vi "CPP-Multiplot.vi"(0 "PlotArray":cluster{dbl[], dbl[]}[](array[cluster]), 1 "Job Directory":path) -> (2 "Saved Automatically?":bool, 3 "gnuplotScript":string, 4 "Plot data file":path)   [LabVIEW 2013]
uses:
  gnuplotScriptComponents/plotstyle.ctl
  gnuplotScriptComponents/graphPeripherals.ctl
  gnuplotScriptComponents/minAndMax.ctl
  gnuplotScriptComponents/AutoManualNumber.ctl
  gnuplotScriptComponents/ticsAndGrids.ctl
  gnuplotScriptComponents/tics.ctl
  gnuplotScriptComponents/grids.ctl
  gnuplotScriptComponents/legendProperties.ctl
  gnuplotScriptComponents/legendAppearance.ctl
  gnuplotScriptComponents/alignment.ctl
  gnuplotScriptComponents/at.ctl
  gnuplotScriptComponents/margins.ctl
  gnuplotScriptComponents/source.ctl
  gnuplotScriptComponents/Master_Legend.ctl
  gnuplotScriptComponents/MasterPeripherals.ctl
  gnuplotScriptComponents/axisName.ctl
  Results_plotter_Global.vi
panel:
  in  "OpenLogfile?":bool
  in  "Show Script Editor?":bool
  in  "Tab Control":T1(tab)=enum."Appearance"
  in  "Each Graph contains:":T2=enum."Series"
  in  "Rows from:":T2=enum."Until done"
  in  "Columns from:":T2=enum."Selector 1"
  in  "Margins":T3={"Top"=2.0, "Bottom"=2.0, "Left"=2.0, "Right"=2.0}
  in  "Height (in)":dbl=7.0 min=0.5 step=0.5 format="%.1f"
  in  "Width (in)":dbl=10.0 min=0.5 step=0.5 format="%.1f"
  in  "nRows":u8=3 min=1
  in  "nCols":u8=3 min=1
  in  "ScaleAdjust":dbl=0.9 min=0.1 max=2.0 step=0.1
  in  "ManualPlotTitles":string[](array[string])
  out "AutoPlotTitles":string[](array[string])
  in  "Individual Plot Titles":bool=TRUE
  in  "Page Title Pre Block":string
  in  "Page Title Post Block":string
  in  "Values to include in Page Title":i32[](listbox)
  in  "Plot Title Offset (characters)":cluster{"horizontal":dbl, "vertical":dbl}
  out "Final Title":string
  in  "Plot Legends Manual":string[](array[string])
  in  "Plotstyles":T4[](array[typedef])=[{"Style"="linespoints", "Color"=16711680, "PointType"=1, "PointSize"=1.0000001, "LineWidth"=1.0, "LineType"=1}, {"Style"="linespoints", "Color"=16860, "PointType"=2, "PointSize"=1.0000001, "LineWidth"=1.0, "LineType"=1}, {"Style"="linespoints", "Color"=51228, "PointType"=3, "PointSize"=1.0, "LineWidth"=1.0, "LineType"=1}, {"Style"="linespoints", "Color"=0, "PointType"=4, "PointSize"=1.0, "LineWidth"=1.0, "LineType"=1}, {"Style"="linespoints", "Color"=9567230, "PointType"=1, "PointSize"=1.0000001, "LineWidth"=1.0, "LineType"=1}, {"Style"="linespoints", "Color"=12369084, "PointType"=1, "PointSize"=1.0000001, "LineWidth"=1.0, "LineType"=1}] caption="Style                      Colour    PointType       PointSize         Linewidth        Linestyle" {"LineType" min=1 max=6 step=1; "LineWidth" min=1 max=6 step=1; "PointSize" min=0 step=0.1}
  out "Plot Legends Auto":string[](array[string])
  out "No of Series supplied":i32
  out "No of Graph Slots Available":i32
  in  "Plot Legends":bool=TRUE
  in  "X axis label":enum32{"Autolabel", "Manual Label"}(tab)
  out "X or theta label":string
  in  "X or theta label Manual":string
  in  "LegendProperties":T5={"Appearance"={"layout"="", "text-sample order"="", "key order"="", "surroundingBox"=""}, "Alignment"={"Horizontal"="", "Vertical"=""}, "Location"="auto", "\"At\" location"={"XcoordSys"="", "YcoordSys"="", "Xvalue"=0.0, "Yvalue"=0.0}}
  in  "Y/R tics And Grids":T9={"tics"={"ticMin"=0.0, "ticStep"=0.0, "ticMax"=0.0, "minorDivsPerMajor"=2, "ticSpacing"=enum."Auto Tics", "ticPosition"=enum."Inside, no mirror"}, "Grids"={"Gridlines"=enum."No grids", "Zeroaxis"=enum."No zero axis"}, "Mapping"=enum."Lin"}
  in  "X/Theta tics And Grids":T9={"tics"={"ticMin"=0.0, "ticStep"=0.0, "ticMax"=0.0, "minorDivsPerMajor"=2, "ticSpacing"=enum."Auto Tics", "ticPosition"=enum."Inside, no mirror"}, "Grids"={"Gridlines"=enum."Major grid", "Zeroaxis"=enum."No zero axis"}, "Mapping"=enum."Lin"}
  in  "PlotType":enum32{"XY", "Polar"}(tab)
  in  "yAxisBounds":T12={"Min"={"Auto"=TRUE, "Value"=0.0}, "Max"={"Auto"=TRUE, "Value"=0.0}}
  in  "Additional XYgnuplot":string
  in  "xAxisBounds":T12={"Min"={"Auto"=TRUE, "Value"=0.0}, "Max"={"Auto"=TRUE, "Value"=0.0}}
  in  "Angle Units":bool=TRUE
  in  "AngleMode":string(combo)="Compass"
  in  "wrapGapsUpTo:":dbl=30.0 step=0.1
  in  "Additional Polar gnuplot":string
  in  "rAxisBounds":T12={"Min"={"Auto"=FALSE, "Value"=0.0}, "Max"={"Auto"=FALSE, "Value"=1.5}}
  in  "Y axis label":enum32{"Autolabel", "Manual Label"}(tab)
  out "Y or R label":string
  in  "Y or R label Manual 2":string
  in  "PeripheralsMasterControl":T14
  in  "Legend Options":T15=enum."Single Legend Below table"
  in  "GraphPeripherals":T16[][](array[typedef])
  out "PlotCommand":string
  in  "Filename Max length":i32=255
  out "File Path Control":path
  out "AuditTrail":string[](array[string])
  out "Desired Legends":string[][](array[string])
  out "original name had conflict":bool
  out "crossplatform problem":bool
  # "Rows/ Columns/ Series from: controls not wired- just a thought for explicit control of what goes where...?"
  # "Overall Page Title"
  # "There are as many graphs as there are titles (from Selector 2)...."
  # "Plot Styles"
  # "Each graph contains plots from Selector 1..."
  # "X/theta"
  # "Y/r"
  # "Shows the numbered line colours and point styles available- well it would, if it didn't disappear every time I update from the repository..!"
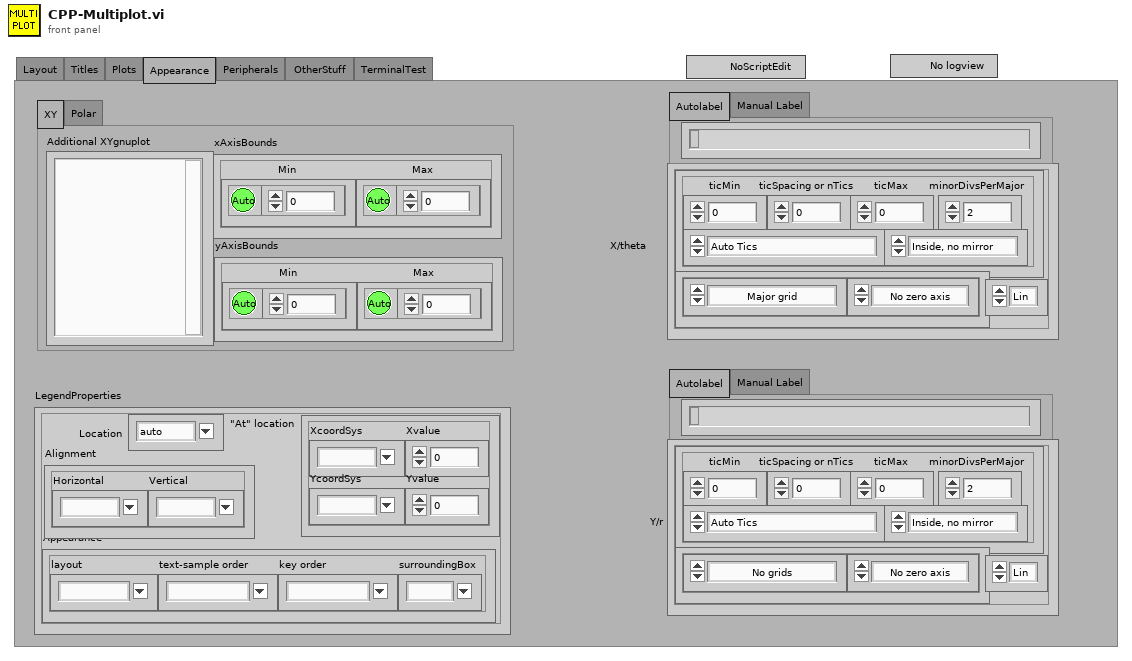
[diagram p1: front panel]
types:
  T1 = enum32{"Layout", "Titles", "Plots", "Appearance", "Peripherals", "OtherStuff ", "TerminalTest"}
  T2 = typedef "source.ctl" = enum16{"Specified:", "Selector 1", "Selector 2", "Until done", "Series"}
  T3 = typedef "margins.ctl" = cluster{"Top":dbl, "Bottom":dbl, "Left":dbl, "Right":dbl}
  T4 = typedef "plotstyle.ctl" = cluster{"Style":string, "Color":u32, "PointType":i32, "PointSize":sgl, "LineWidth":sgl, "LineType":u8}
  T5 = typedef "legendProperties.ctl" = cluster{"Appearance":T6, "Alignment":T7, "Location":string, "\"At\" location":T8}
  T6 = typedef "legendAppearance.ctl" = cluster{"layout":string, "text-sample order":string, "key order":string, "surroundingBox":string}
  T7 = typedef "alignment.ctl" = cluster{"Horizontal":string, "Vertical":string}
  T8 = typedef "at.ctl" = cluster{"XcoordSys":string, "YcoordSys":string, "Xvalue":dbl, "Yvalue":dbl}
  T9 = typedef "ticsAndGrids.ctl" = cluster{"tics":T10, "Grids":T11, "Mapping":enum8{"Lin", "Log"}}
  T10 = typedef "tics.ctl" = cluster{"ticMin":dbl, "ticStep":dbl, "ticMax":dbl, "minorDivsPerMajor":i32, "ticSpacing":enum16{"Auto Tics", "Fixed spacing", "Fixed Minimum and Spacing", "Start, Spacing and Maximum", "Approx n Tics (rounded)"}, "ticPosition":enum16{"Inside, no mirror", "Inside, mirrored", "Outside, no mirror", "Outside, mirrored", "Invisible"}}
  T11 = typedef "grids.ctl" = cluster{"Gridlines":enum16{"No grids", "Major grid", "Minor grid", "Major and Minor"}, "Zeroaxis":enum16{"No zero axis", "Show zero axis"}}
  T12 = typedef "minAndMax.ctl" = cluster{"Min":T13, "Max":T13}
  T13 = typedef "AutoManualNumber.ctl" = cluster{"Auto":bool, "Value":dbl}
  T14 = typedef "MasterPeripherals.ctl" = enum16{"Use Table", "Titles On", "Edges Only", "All Off"}
  T15 = typedef "Master_Legend.ctl" = enum16{"No Legend", "Single Legend Below table", "Legend as per array"}
  T16 = typedef "graphPeripherals.ctl" = cluster{"title":bool, "key":bool, "Xtic":bool, "Ytic":bool, "Xlab":bool, "Ylab":bool}
  T17 = typedef "axisName.ctl" = string
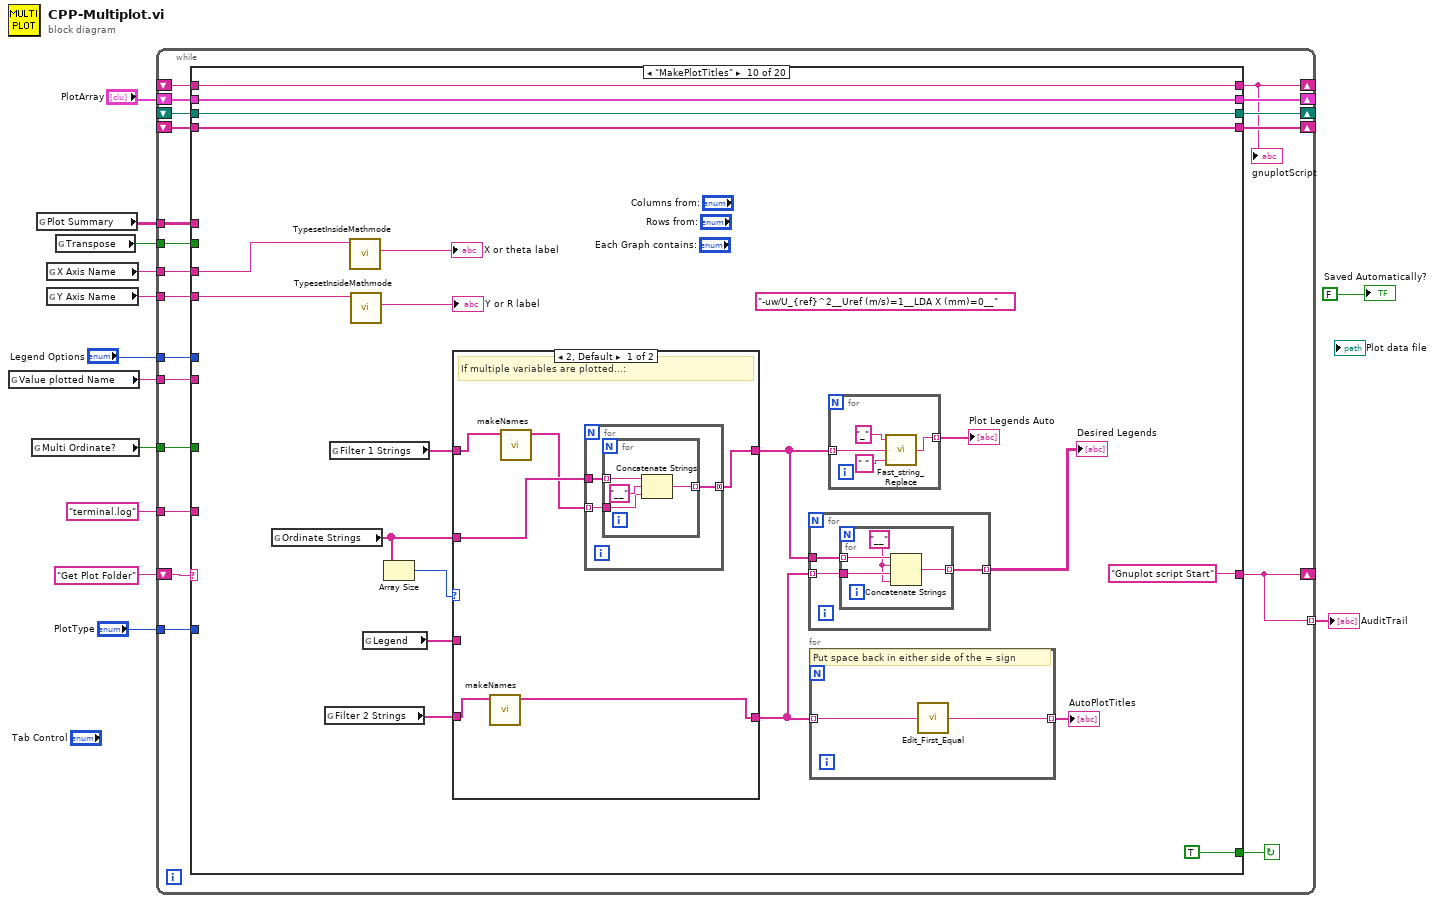
[diagram p0: block diagram]
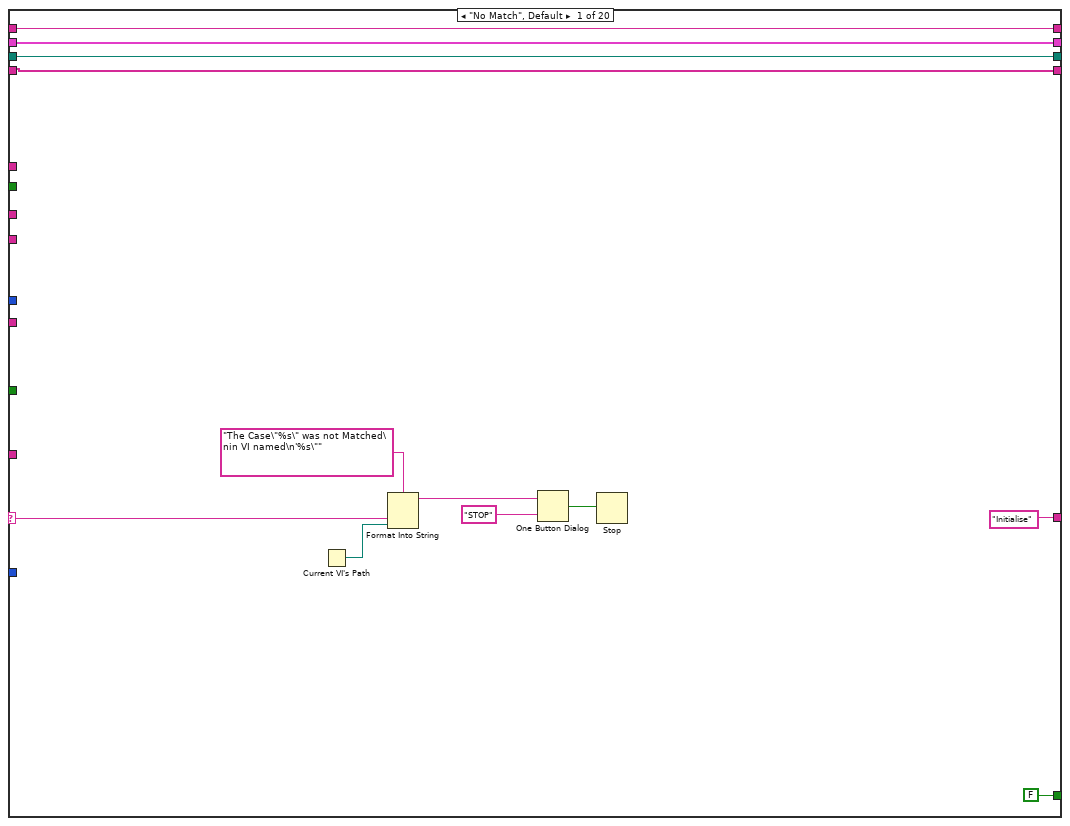
[diagram p2: hidden frame]
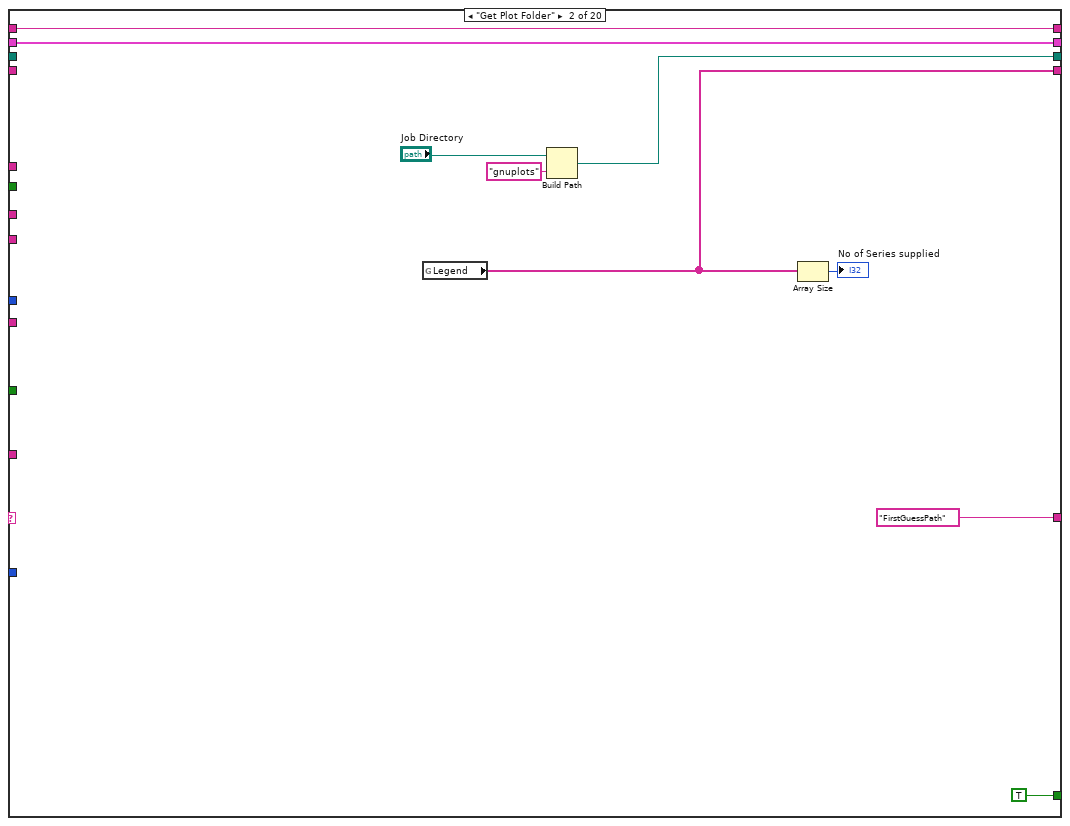
[diagram p3: hidden frame]
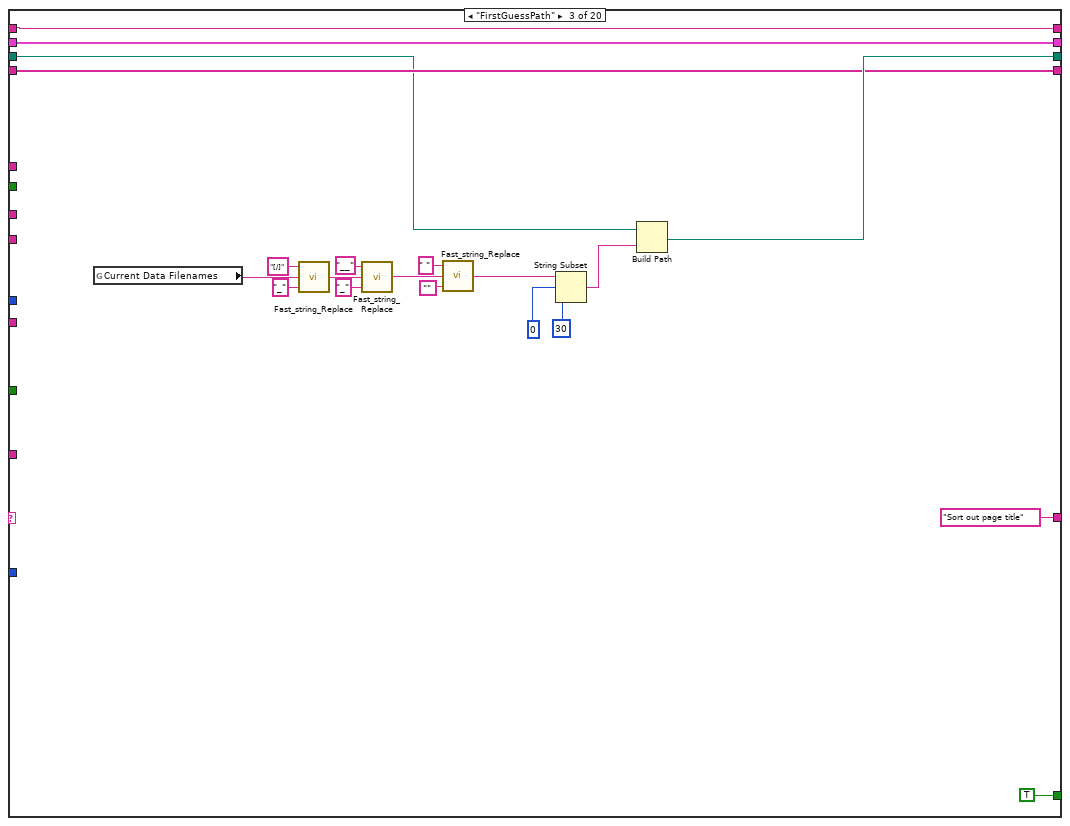
[diagram p4: hidden frame]
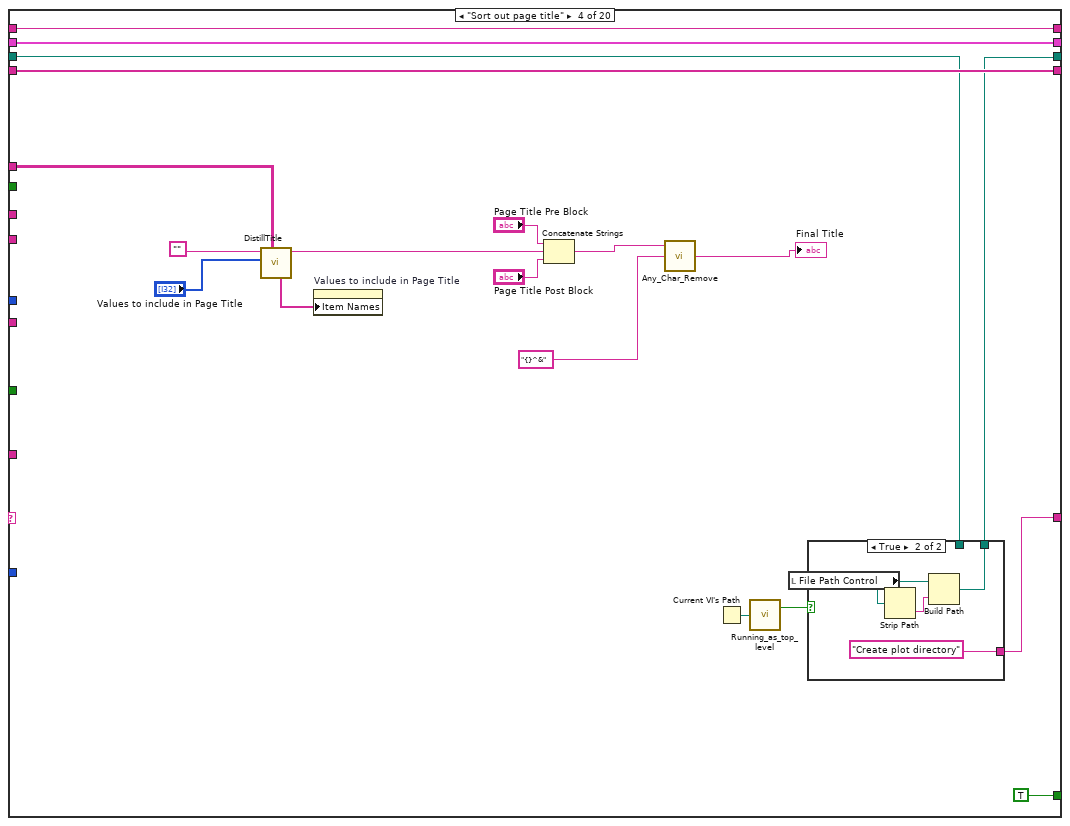
[diagram p5: hidden frame]
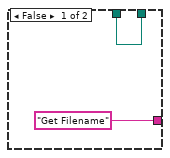
[diagram p6: hidden frame]
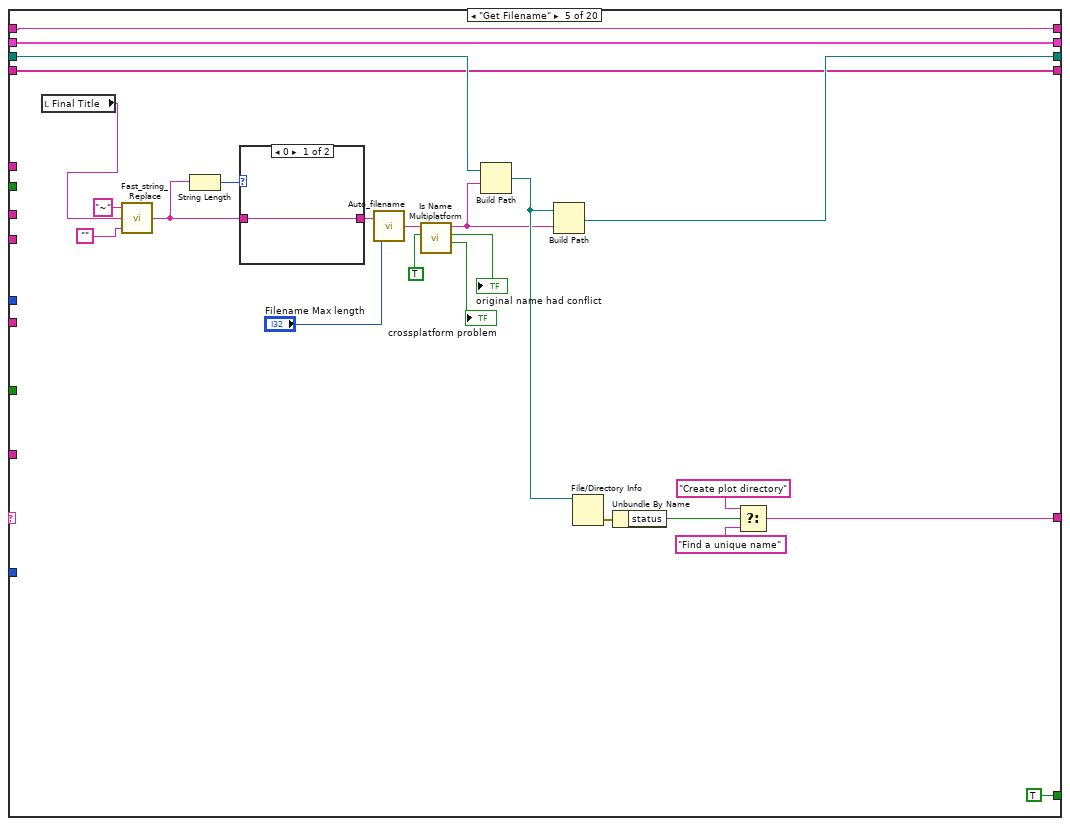
[diagram p7: hidden frame]
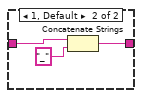
[diagram p8: hidden frame]
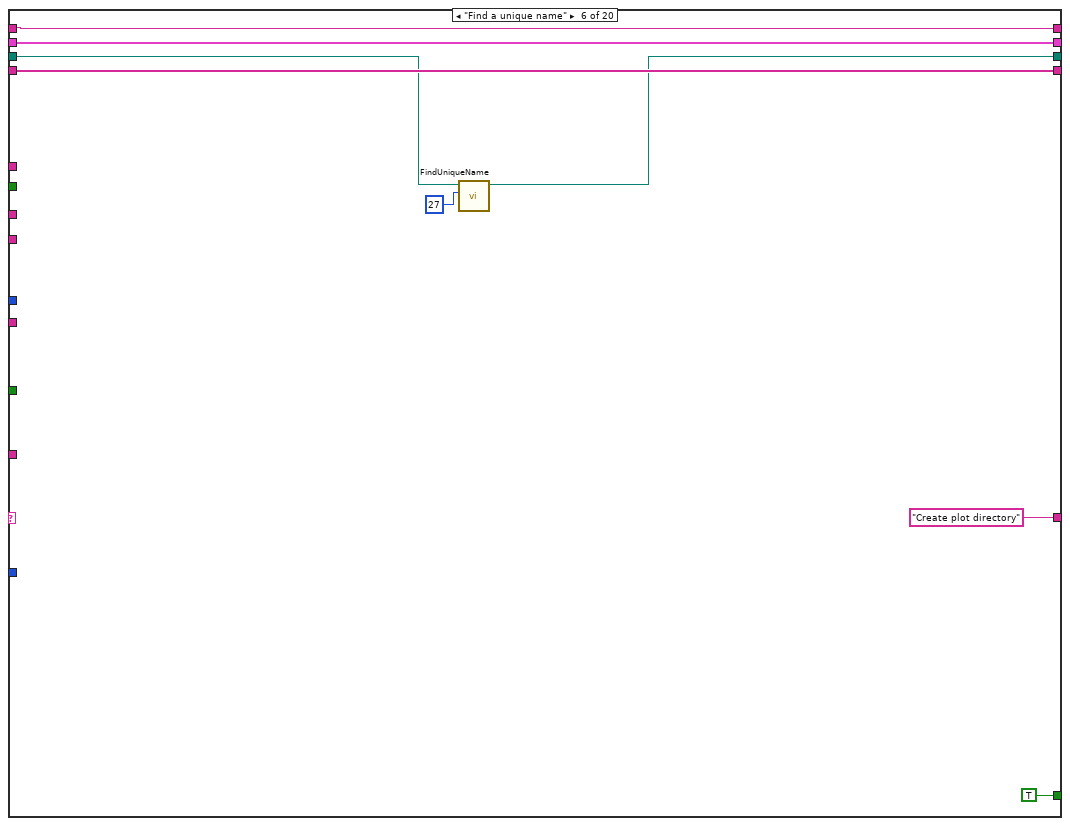
[diagram p9: hidden frame]
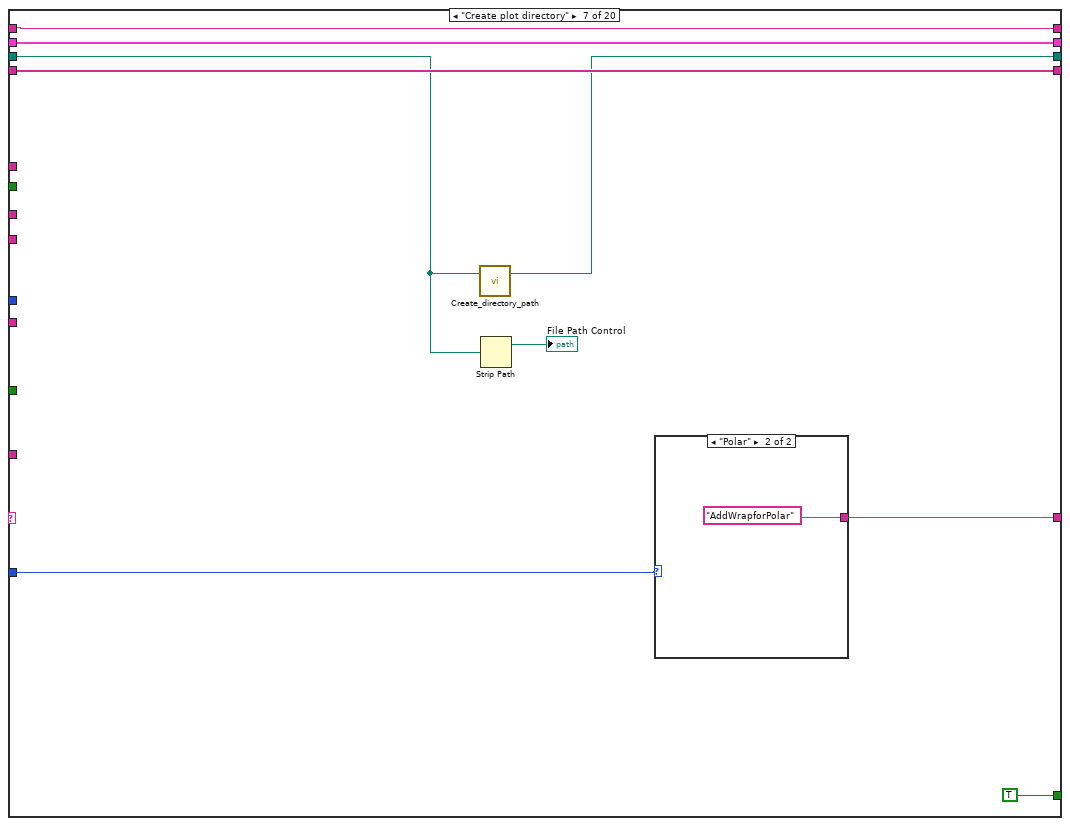
[diagram p10: hidden frame]
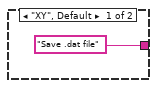
[diagram p11: hidden frame]
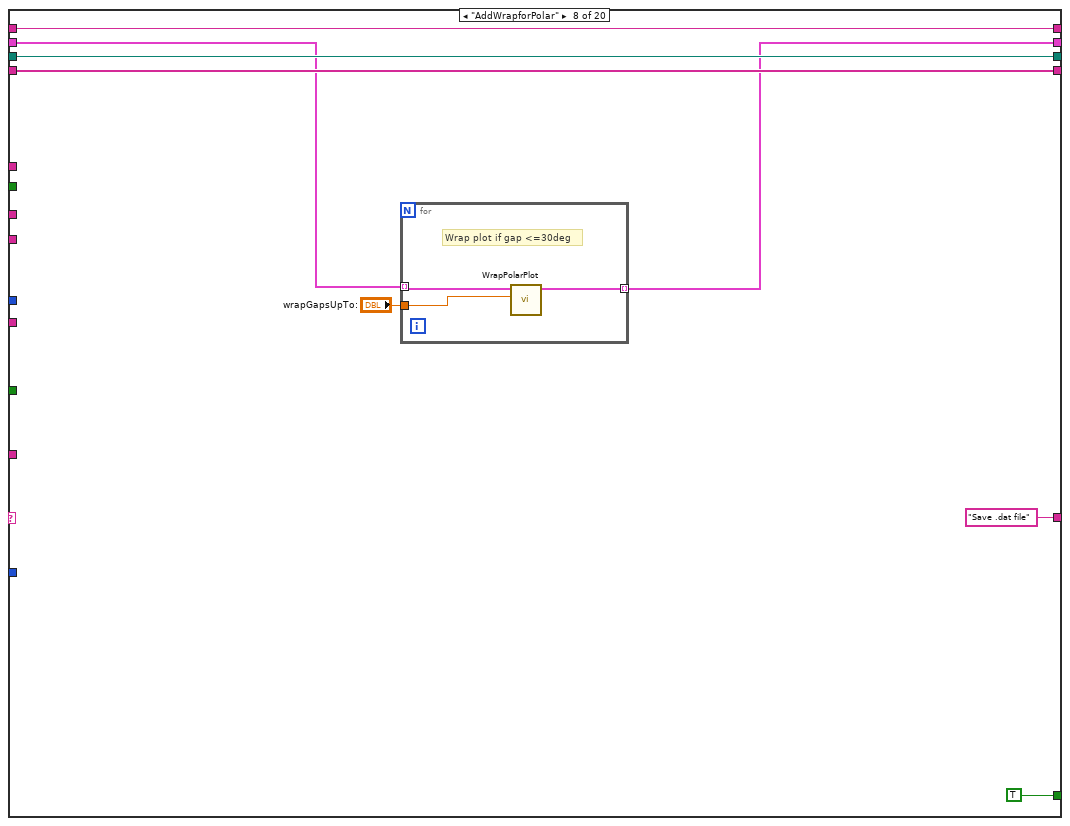
[diagram p12: hidden frame]
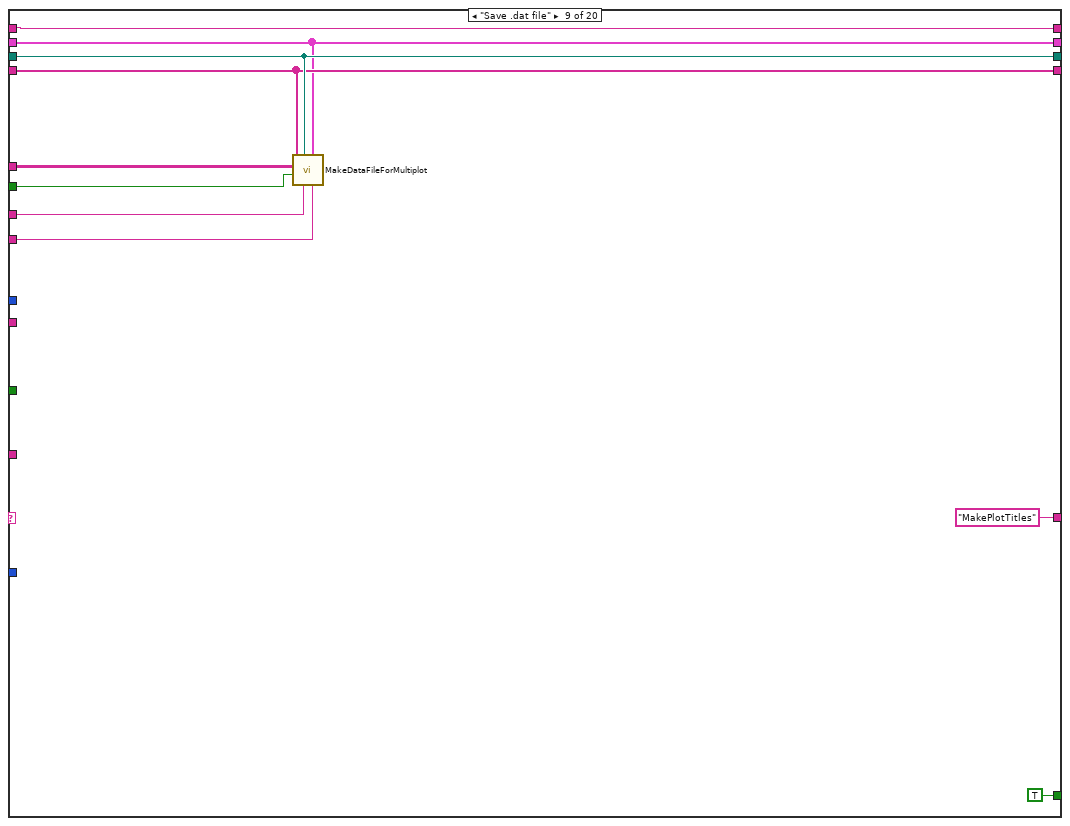
[diagram p13: hidden frame]
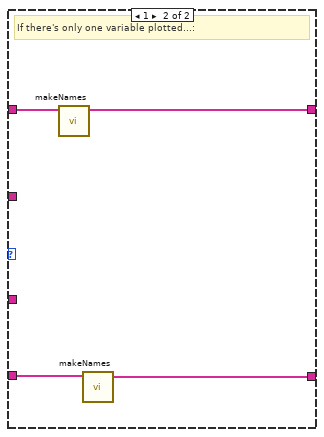
[diagram p14: hidden frame]
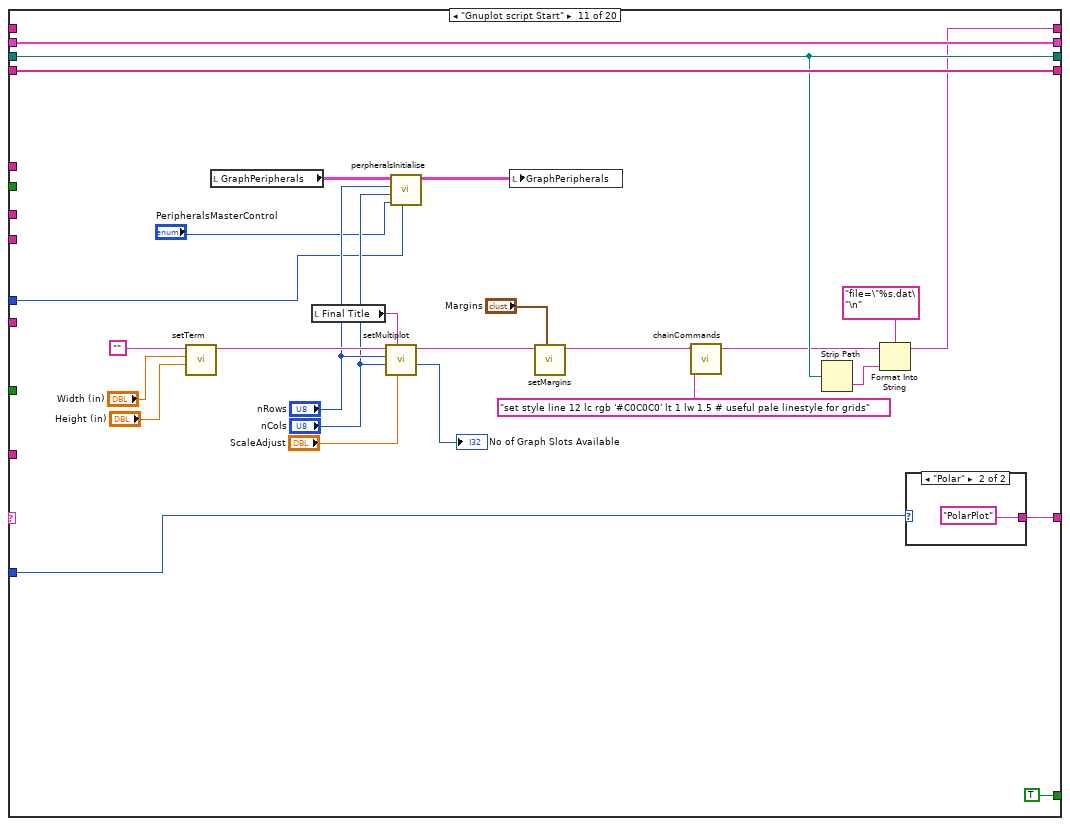
[diagram p15: hidden frame]
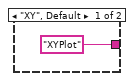
[diagram p16: hidden frame]
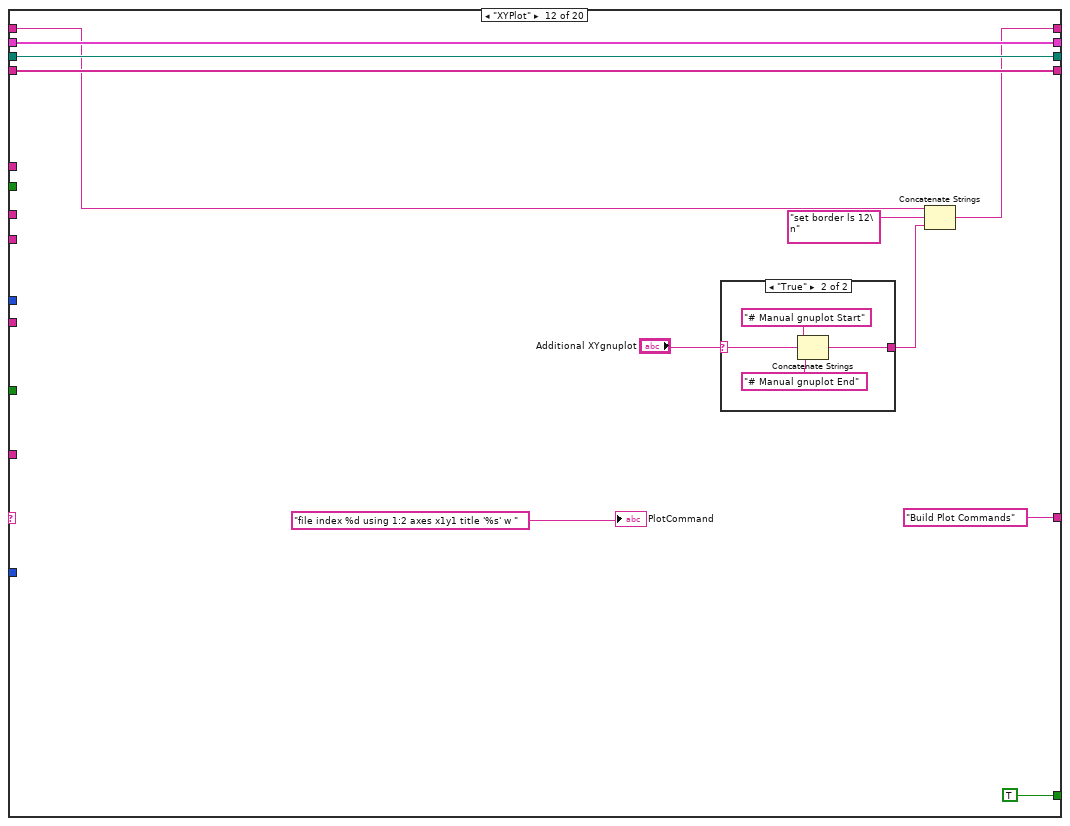
[diagram p17: hidden frame]
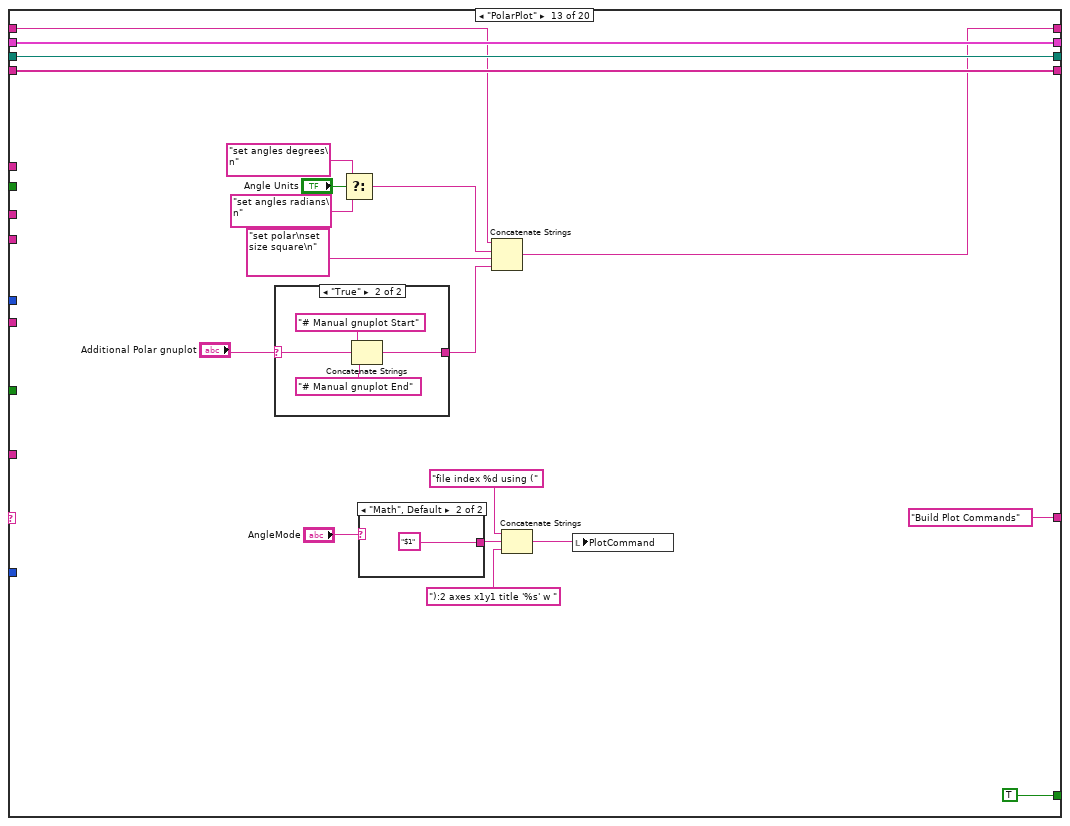
[diagram p19: hidden frame]
diagram:
  n1 = global read "Results_plotter_Global.vi" "Value plotted Name"() -> (w9:string)
  n2 = global read "Results_plotter_Global.vi" "Multi Ordinate?"() -> (w5:bool)
  n3 = global read "Results_plotter_Global.vi" "Plot Summary"() -> (w12:string[][])
  n4 = global read "Results_plotter_Global.vi" "X Axis Name"() -> (w11:string)
  n5 = global read "Results_plotter_Global.vi" "Y Axis Name"() -> (w10:string)
  n6 = global read "Results_plotter_Global.vi" "Transpose"() -> (w6:bool)
  n7 = while {
    shift-left: "Get Plot Folder" -> [w32]
    shift-right: [w16] -> _
    tunnel: w12 -> [w31]
    shift-right: [w30] -> _
    shift-left: _ -> [w29]
    tunnel: w11 -> [w28]
    tunnel: w10 -> [w27]
    tunnel: w9 -> [w26]
    shift-right: [w24] -> _
    shift-left: "PlotArray" -> [w25]
    shift-right: [w17] -> _
    shift-left: _ -> [w23]
    shift-right: [w22] -> _
    shift-left: _ -> [w21]
    tunnel: "terminal.log" -> [w20]
    tunnel: w6 -> [w19]
    tunnel: w5 -> [w18]
    tunnel: [w16] -> w4 mode=indexing
    tunnel: "PlotType" -> [w15]
    tunnel: "Legend Options" -> [w14]
    stop <- w33 continue-if-true
    n8 = case shown="\"MakePlotTitles\"" w32 {
      selector: w32 -> [w34 _ _ _ _ _ _ _ _ _ _ _ _ _ _ _ _ _ _ _]
      tunnel: [FALSE TRUE TRUE ("Top Level") TRUE ("Top Level") TRUE ("Top Level") TRUE ("Top Level") TRUE TRUE ("Top Level") TRUE ("Top Level") TRUE ("Top Level") TRUE ("Top Level") TRUE ("Top Level") TRUE ("Top Level") TRUE ("Top Level") TRUE ("Top Level") TRUE ("Top Level") TRUE ("Top Level") FALSE ("Top Level") TRUE ("Top Level") FALSE ("Top Level")] -> w33
      tunnel: ["Initialise" "FirstGuessPath" "Sort out page title" w85 w121 "Create plot directory" w136 "Save .dat file" "MakePlotTitles" "Gnuplot script Start" w241 "Build Plot Commands" "Build Plot Commands" "Write gnuplot file" ("t") "Execute shell script" ("t") "Has pdf been generated?" ("t") w429 "End" "End" ("t") "End" ("t")] -> w16
      tunnel: w31 -> [_ _ _ w80 _ _ _ _ w165 _ _ _ _ _ _ _ _ _ _ _]
      tunnel: [w38 w52 w74 w87 w122 w128 w141 w153 w166 w187 w232 w257 w280 w326 w411 w419 w433 w438 w448 w459] -> w30
      tunnel: w29 -> [w38 _ w70 w86 w118 w129 w140 w153 w166 w187 w232 w257 w280 w326 w411 w419 w433 w438 w448 w459]
      tunnel: w28 -> [_ _ _ _ _ _ _ _ w164 w180 _ _ _ _ _ _ _ _ _ _]
      tunnel: w27 -> [_ _ _ _ _ _ _ _ w163 w179 _ _ _ _ _ _ _ _ _ _]
      tunnel: w26 -> [_ _ _ _ _ _ _ _ _ _ _ _ _ _ _ _ _ _ _ _]
      tunnel: w25 -> [w37 w48 w73 w93 w120 w132 w144 w149 w160 w186 w244 w256 w281 w291 w417 w424 w436 w443 w453 w458]
      tunnel: [w37 w48 w73 w93 w120 w132 w144 w148 w160 w186 w244 w256 w281 w291 w417 w424 w436 w443 w453 w458] -> w24
      tunnel: w23 -> [w36 w51 w72 w91 w119 w131 w143 w154 w167 w185 _ w249 w275 w318 w407 w422 w434 w441 w451 w457]
      tunnel: [w36 w51 w72 w91 w119 w131 w143 w154 w167 w185 w229 w252 w276 w324 w407 w422 w434 w441 w451 w457] -> w17
      tunnel: [w35 w47 w71 w92 w117 w130 w142 w152 w162 w184 w243 w255 w279 w325 w412 w423 w435 w442 w452 w456] -> w22
      tunnel: w21 -> [w35 _ w71 w92 w117 w130 w142 w152 w162 w184 w243 w255 w279 w325 w412 w423 w435 w442 w452 w456]
      tunnel: w20 -> [_ _ _ _ _ _ _ _ _ _ _ _ _ _ _ w418 _ _ w446 _]
      tunnel: w19 -> [_ _ _ _ _ _ _ _ w161 _ _ _ _ _ _ _ _ _ _ _]
      tunnel: w18 -> [_ _ _ _ _ _ _ _ _ _ _ _ _ _ _ _ _ _ _ _]
      tunnel: w15 -> [_ _ _ _ _ _ w137 _ _ _ w228 _ _ w304 _ _ _ _ _ _]
      tunnel: w14 -> [_ _ _ _ _ _ _ _ _ _ w219 _ _ w290 _ _ _ _ _ _]
      frame "No Match", Default {
        n9 = Current VI's Path() -> (path=w40:path)
        n10 = Format Into String(format string="The Case\"%s\" was not Matched\nin VI named\n'%s\"" ("Format String"), w34, w40) -> (resulting string=w43:string)  [unwired: 2 in, 1 out]
        n11 = One Button Dialog(message=w43, button name ("OK")="STOP") -> (true=w41:bool)
        n12 = Stop(stop? (T)=w41) -> ()
      }
      frame "Get Plot Folder" {
        n13 = global read "Results_plotter_Global.vi" "Legend"() -> (w47:string[])
        n14 = Build Path(base path="Job Directory", name or relative path="gnuplots") -> (appended path=w52:path)
        n15 = Array Size(array=w47) -> (size(s)=→"No of Series supplied":i32)
      }
      frame "FirstGuessPath" {
        n16 = global read "Results_plotter_Global.vi" "Current Data Filenames"() -> (w59:string)
        n17 = call "Fast_string_Replace.vi"("Replace match with:"="_", "Input String"=w59, "regular expression"="[/]") -> ("Output String"=w63:string)  [unwired: 2 out]
        n18 = call "Fast_string_Replace.vi"("Replace match with:"="_", "Input String"=w63, "regular expression"="__") -> ("Output String"=w60:string)  [unwired: 2 out]
        n19 = call "Fast_string_Replace.vi"("Replace match with:"="", "Input String"=w60, "regular expression"=" ") -> ("Output String"=w58:string)  [unwired: 2 out]
        n20 = String Subset(string=w58, offset (0)=0, length (rest)=30 ("length (rest)")) -> (substring=w57:string)
        n21 = Build Path(base path=w70, name or relative path=w57) -> (appended path=w74:path)
      }
      frame "Sort out page title" {
        n22 = call "DistillTitle.vi"("Plot Summary in"=w80, "Indices to include in Page Title"="Values to include in Page Title", "String in"="") -> ("String out"=w84:string, "AvailableVariables"=w78:string[])  [unwired: 7 in]
        n23 = property on="Values to include in Page Title" class="LstBox (strict)"("Item Names"=w78) -> ()  [unwired: 2 in, 2 out]
        n24 = Concatenate Strings("Page Title Pre Block", w84, "Page Title Post Block") -> (w77:string)
        n25 = call "Any_Char_Remove.vi"("Individual Characters to Remove"="{}^&", "String in"=w77) -> ("String out"=→"Final Title":string)  [unwired: 1 in]
        n26 = Current VI's Path() -> (path=w90:path)
        n27 = call "Running_as_top_level.vi"("Vi path name"=w90) -> ("Top Level"=w88:bool)  [unwired: 1 out]
        n28 = case shown="True" w88 {
          tunnel: [w95 w98] -> w87
          tunnel: w86 -> [w95 _]
          tunnel: ["Get Filename" ("t") "Create plot directory"] -> w85
          frame False {
          }
          frame True {
            n29 = local read "File Path Control"() -> (w97:path)
            n30 = Strip Path(path=w97) -> (name=w96:string)  [unwired: 1 out]
            n31 = Build Path(base path=w97, name or relative path=w96) -> (appended path=w98:path)
          }
        }
      }
      frame "Get Filename" {
        n32 = local read "Final Title"() -> (w107:string)
        n33 = call "Fast_string_Replace.vi"("Replace match with:"="", "Input String"=w107, "regular expression"="~") -> ("Output String"=w104:string)  [unwired: 1 in, 1 out]
        n34 = String Length(string=w104) -> (length=w109:i32)
        n35 = case shown="0" w109 {
          tunnel: [w124 w125] -> w108
          tunnel: w104 -> [w124 w127]
          frame 0 {
          }
          frame 1, Default {
            n36 = Concatenate Strings(w127, "_") -> (w125:string)
          }
        }
        n37 = call "Auto_filename.vi"("Filename Max length"="Filename Max length", "Prefix"=w108) -> ("Filename"=w111:string)
        n38 = call <vilib>:"Is Name Multiplatform.vi"("name must work for all platforms (F)"=TRUE, "filename"=w111) -> ("crossplatform problem"=→"crossplatform problem":bool, "original name had conflict"=→"original name had conflict":bool, "suggested filename"=w103:string)  [unwired: 5 in, 2 out]
        n39 = Build Path(base path=w118, name or relative path=w103) -> (appended path=w115:path)
        n40 = Build Path(base path=w115, name or relative path=w103) -> (appended path=w122:path)
        n41 = File/Directory Info(path=w115) -> (error out=w116:errorcluster)  [unwired: 1 in, 6 out]
        n42 = Unbundle By Name(w116) -> ("status"=w114:bool)
        n43 = Select(t="Create plot directory", s=w114, f="Find a unique name") -> (s? t:f=w121:string)
      }
      frame "Find a unique name" {
        n44 = call "FindUniqueName.vi"("Max Length"=27, "PathIn"=w129) -> ("UniquedPath"=w128:path)  [unwired: 9 in]
      }
      frame "Create plot directory" {
        n45 = call "Create_directory_path.vi"("Path name"=w140) -> ("Path name Out"=w141:path)  [unwired: 1 in, 1 out]
        n46 = Strip Path(path=w140) -> (stripped path=→"File Path Control":path)  [unwired: 1 out]
        n47 = case shown="\"Polar\"" w137 {
          tunnel: ["Save .dat file" "AddWrapforPolar"] -> w136
          frame "XY", Default {
          }
          frame "Polar" {
          }
        }
      }
      frame "AddWrapforPolar" {
        n48 = for {
          tunnel: w149 -> [w157] mode=indexing
          tunnel: [w156] -> w148 mode=indexing
          tunnel: "wrapGapsUpTo:" -> [w155]
          # "Wrap plot if gap <=30deg"
          n49 = call "WrapPolarPlot.vi"("maxWrap"=w155, "thetaRin"=w157) -> ("thetaRout"=w156:cluster{"Angle":dbl[], "Radius":dbl[]})  [unwired: 9 in]
        }
      }
      frame "Save .dat file" {
        n50 = call "MakeDataFileForMultiplot.vi"("Y Axis Name"=w163, "Plot Array"=w160, "X Axis Name"=w164, "Path"=w166, "Transpose"=w161, "Plot Summary"=w165, "Legend"=w162) -> ()  [unwired: 5 in]
      }
      frame "MakePlotTitles" {
        (unwired) "-uw/U_{ref}^2__Uref (m/s)=1__LDA X (mm)=0__"
        n51 = global read "Results_plotter_Global.vi" "Ordinate Strings"() -> (w171:string[])
        n52 = global read "Results_plotter_Global.vi" "Filter 2 Strings"() -> (w176:string[])
        n53 = global read "Results_plotter_Global.vi" "Filter 1 Strings"() -> (w177:string[])
        n54 = call "TypesetInsideMathmode.vi"("DirtyString"=w180) -> ("Mathmode String"=→"X or theta label":string)  [unwired: 9 in, 1 out]
        n55 = call "TypesetInsideMathmode.vi"("DirtyString"=w179) -> ("Mathmode String"=→"Y or R label":string)  [unwired: 9 in, 1 out]
        n56 = global read "Results_plotter_Global.vi" "Legend"() -> (w182:string[])
        n57 = Array Size(array=w171) -> (size(s)=w170:i32)
        n58 = case shown="2, Default" w170 {
          tunnel: w182 -> [_ _]
          tunnel: [w204 w216] -> w175
          tunnel: [w201 w214] -> w169
          tunnel: w171 -> [w203 _]
          tunnel: w177 -> [w206 w217]
          tunnel: w176 -> [w205 w215]
          frame 2, Default {
            # "If multiple variables are plotted...:"
            n59 = call "makeNames.vi"("Strings"=w205) -> ("Names"=w204:string[])  [unwired: 10 in]
            n60 = call "makeNames.vi"("Strings"=w206) -> ("Names"=w202:string[])  [unwired: 10 in]
            n61 = for {
              tunnel: w203 -> [w209]
              tunnel: w202 -> [w208] mode=indexing
              tunnel: [w207] -> w201 mode=concatenating
              n62 = for {
                tunnel: w209 -> [w213] mode=indexing
                tunnel: w208 -> [w211]
                tunnel: [w210] -> w207 mode=indexing
                n63 = Concatenate Strings(w213, "__" ("string"), w211) -> (w210:string)
              }
            }
          }
          frame 1 {
            # "If there's only one variable plotted...:"
            n64 = call "makeNames.vi"("Strings"=w217) -> ("Names"=w214:string[])  [unwired: 10 in]
            n65 = call "makeNames.vi"("Strings"=w215) -> ("Names"=w216:string[])  [unwired: 10 in]
          }
        }
        n66 = for {
          tunnel: w169 -> [w196]
          tunnel: w175 -> [w195] mode=indexing
          tunnel: [w194] -> w178 mode=indexing
          n67 = for {
            tunnel: w196 -> [w200] mode=indexing
            tunnel: w195 -> [w199]
            tunnel: [w197] -> w194 mode=indexing
            w198 = "__" ("string")
            n68 = Concatenate Strings(w200, w198, w199, w198) -> (w197:string)
          }
        }
        "Desired Legends" <- w178
        n69 = for {
          tunnel: w175 -> [w193] mode=indexing
          tunnel: [w192] -> w174 mode=indexing
          # "Put space back in either side of the = sign"
          n70 = call "Edit_First_Equal.vi"("String in"=w193) -> ("String out"=w192:string)
        }
        "AutoPlotTitles" <- w174
        n71 = for {
          tunnel: w169 -> [w189] mode=indexing
          tunnel: [w188] -> w168 mode=indexing
          n72 = call "Fast_string_Replace.vi"("Replace match with:"=" ", "Input String"=w189, "regular expression"="_") -> ("Output String"=w188:string)  [unwired: 2 out]
        }
        "Plot Legends Auto" <- w168
      }
      frame "Gnuplot script Start" {
        n73 = call "setTerm.vi"("Height (in)"="Height (in)", "Width (in)"="Width (in)", "String in"="") -> ("String out"=w237:string)  [unwired: 7 in, 1 out]
        n74 = local read "GraphPeripherals"() -> (w224:T16[][])
        n75 = local read "Final Title"() -> (w235:string)
        n76 = call "setMultiplot.vi"("ScaleAdjust"="ScaleAdjust", "OverallTitle"=w235, "Cols"="nCols", "Rows"="nRows", "String in"=w237) -> ("nGraphs"=→"No of Graph Slots Available":i32, "String out"=w236:string)  [unwired: 4 in, 1 out]
        n77 = call "perpheralsInitialise.vi"("Legend"=w219, "PeripheralsMasterControl"="PeripheralsMasterControl", "Cols"="nCols", "Rows"="nRows", "GraphPeripheralsIn"=w224) -> ("GraphPeripheralsOut"=w225:T16[][])  [unwired: 6 in]
        n78 = local write "GraphPeripherals"(w225) -> ()
        n79 = call "setMargins.vi"("Margins"="Margins", "String in"=w236) -> ("String out"=w221:string)  [unwired: 8 in, 1 out]
        n80 = call "chainCommands.vi"("Command"="set style line 12 lc rgb '#C0C0C0' lt 1 lw 1.5 # useful pale linestyle for grids", "StringIn"=w221) -> ("StringOut"=w222:string)  [unwired: 9 in]
        n81 = Strip Path(path=w232) -> (name=w231:string)  [unwired: 1 out]
        n82 = Format Into String(format string="file=\"%s.dat\"\n" ("string"), initial string=w222, w231) -> (resulting string=w229:string)  [unwired: 1 in, 1 out]
        n83 = case shown="\"Polar\"" w228 {
          tunnel: ["XYPlot" "PolarPlot"] -> w241
          frame "XY", Default {
          }
          frame "Polar" {
          }
        }
      }
      frame "XYPlot" {
        n84 = case shown="\"True\"" "Additional XYgnuplot" {
          selector: "Additional XYgnuplot" -> [w258 w262]
          tunnel: [w258 w261] -> w247
          frame "", Default {
          }
          frame "True" {
            n85 = Concatenate Strings("# Manual gnuplot Start" ("string"), w262, "# Manual gnuplot End" ("string")) -> (w261:string)
          }
        }
        n86 = Concatenate Strings(w249, "set border ls 12\n" ("input 2"), w247) -> (w252:string)
        "PlotCommand" <- "file index %d using 1:2 axes x1y1 title '%s' w " ("format string")
      }
      frame "PolarPlot" {
        n87 = case shown="\"True\"" "Additional Polar gnuplot" {
          selector: "Additional Polar gnuplot" -> [w282 w286]
          tunnel: [w282 w285] -> w263
          frame "", Default {
          }
          frame "True" {
            n88 = Concatenate Strings("# Manual gnuplot Start" ("string"), w286, "# Manual gnuplot End" ("string")) -> (w285:string)
          }
        }
        n89 = Select(t="set angles degrees\n", s="Angle Units", f="set angles radians\n") -> (s? t:f=w265:string)
        n90 = case shown="\"Math\", Default" "AngleMode" {
          tunnel: ["90-$1" ("format string") "$1" ("format string")] -> w270
          frame "Compass" {
          }
          frame "Math", Default {
          }
        }
        n91 = Concatenate Strings(w275, w265, "set polar\nset size square\n", w263) -> (w276:string)
        n92 = Concatenate Strings("file index %d using (" ("format string"), w270, "):2 axes x1y1 title '%s' w " ("format string")) -> (w269:string)
        n93 = local write "PlotCommand"(w269) -> ()
      }
      frame "Build Plot Commands" {
        n94 = local read "Plot Legends Auto"() -> (w293:string[])
        n95 = local read "AutoPlotTitles"() -> (w316:string[])
        n96 = case shown="\"Autolabel\", Default" "Y axis label" {
          tunnel: [w327 "Y or R label Manual 2"] -> w299
          frame "Autolabel", Default {
            n97 = local read "Y or R label"() -> (w327:string)
          }
          frame "Manual Label" {
          }
        }
        n98 = case shown="\"Autolabel\", Default" "X axis label" {
          tunnel: [w335 "X or theta label Manual"] -> w305
          frame "Autolabel", Default {
            n99 = local read "X or theta label"() -> (w335:string)
          }
          frame "Manual Label" {
          }
        }
        n100 = Select(t=w293, s="Plot Legends", f="Plot Legends Manual") -> (s? t:f=w292:string[])
        n101 = local read "Desired Legends"() -> (w312:string[][])
        n102 = local read "PlotCommand"() -> (w307:string)
        n103 = case shown="Default" w304 {
          tunnel: [T17 "theta" ("Axis") T17 "x" ("Axis")] -> w302
          tunnel: [T17 "r" ("Axis") T17 "y" ("Axis")] -> w301
          tunnel: ["rAxisBounds" "yAxisBounds"] -> w303
          frame "Polar" {
          }
          frame Default {
          }
        }
        n104 = global read "Results_plotter_Global.vi" "Legend"() -> (w311:string[])
        n105 = call "serialiseArray.vi"("GraphPeripherals"="GraphPeripherals") -> ("output array"=w313:T16[])  [unwired: 10 in]
        n106 = Select(t=w316, s="Individual Plot Titles", f="ManualPlotTitles") -> (s? t:f=w289:string[])
        n107 = for {
          shift-right: [w359] -> w319
          shift-left: "\n#Begin plots\n" -> [w357]
          tunnel: w292 -> [w360]
          tunnel: "Plotstyles" -> [w361]
          tunnel: w289 -> [w353] mode=indexing
          tunnel: w313 -> [w356] mode=indexing
          tunnel: w312 -> [w355] mode=indexing
          tunnel: w311 -> [w354]
          tunnel: "LegendProperties" -> [w341]
          tunnel: "Plot Title Offset (characters)" -> [w352]
          tunnel: w307 -> [w351]
          tunnel: w305 -> [w350]
          tunnel: w303 -> [w349]
          tunnel: w302 -> [w348]
          tunnel: w301 -> [w347]
          tunnel: w299 -> [w346]
          tunnel: "Y/R tics And Grids" -> [w345]
          tunnel: "X/Theta tics And Grids" -> [w344]
          tunnel: "xAxisBounds" -> [w343]
          tunnel: w291 -> [w342]
          tunnel: w290 -> [w340]
          i -> [w339]
          # "Loops once for each graph on the multiplot"
          n108 = call "BuildPlotsOneGraph.vi"("Legend"=w354, "Desired Legends"=w355, "PlotArray"=w342, "Plot Legends"=w360, "Plotstyles"=w361, "PlotCommand"=w351) -> ("Yspan"=w338:cluster{"Max":dbl, "Min":dbl}, "Xspan"=w337:cluster{"Max":dbl, "Min":dbl}, "String out"=w358:string)  [unwired: 1 in, 2 out]
          n109 = stacked-sequence {
            seq-local: [w367 _] -> [_ w384]
            seq-local: [w363 _] -> [_ w383]
            tunnel: [_ w406] -> w359
            tunnel: w358 -> [_ w405]
            tunnel: w357 -> [_ w404]
            tunnel: w356 -> [w365 w403]
            tunnel: w353 -> [_ w394]
            tunnel: w352 -> [_ w392]
            tunnel: w350 -> [_ w391]
            tunnel: w349 -> [_ w382]
            tunnel: w348 -> [_ w390]
            tunnel: w347 -> [_ w389]
            tunnel: w346 -> [_ w388]
            tunnel: w345 -> [_ w387]
            tunnel: w344 -> [_ w386]
            tunnel: w343 -> [_ w381]
            tunnel: w341 -> [w366 _]
            tunnel: w340 -> [w368 _]
            tunnel: w339 -> [w362 _]
            tunnel: w338 -> [_ w379]
            tunnel: w337 -> [_ w380]
            frame #0 {
              n110 = Unbundle By Name(w365) -> ("key"=w364:bool)
              n111 = case shown="\"Single Legend Below table\"" w368 {
                tunnel: [w370 w372] -> w367
                tunnel: w366 -> [w370 w378]
                tunnel: w364 -> [w369 _]
                tunnel: [w369 w371] -> w363
                tunnel: w362 -> [_ w373]
                frame "Legend as per array", Default {
                }
                frame "Single Legend Below table" {
                  w376 = "screen" ("\"At\" location.XcoordSys")
                  # "Use \"screen\" coordinates to place legend at bottom-center\nof entire \"screen\" of graphs; update legend cluster to \nreflect this."
                  # "Only legend the first graph"
                  n112 = Equal To 0?(x=w373) -> (x = 0?=w371:bool)
                  n113 = Bundle By Name(cluster=w378, "Location"="at", "\"At\" location.XcoordSys"=w376, "\"At\" location.Xvalue"=0.6 ("\"At\" location.Xvalue"), "\"At\" location.YcoordSys"=w376, "\"At\" location.Yvalue"=-0.03 ("\"At\" location.Yvalue")) -> (w372:T5)
                  n114 = local write "LegendProperties"(w372) -> ()
                }
              }
            }
            frame #1 {
              n115 = Unbundle By Name(w403) -> ("title"=w402:bool, "Xtic"=w398:bool, "Xlab"=w397:bool, "Ytic"=w396:bool, "Ylab"=w395:bool)
              n116 = call "TypesetInsideMathmode.vi"("DirtyString"=w394) -> ("Mathmode String"=w385:string)  [unwired: 9 in, 1 out]
              n117 = call "setTitle.vi"("Offset"=w392, "Set?"=w402, "Title"=w385, "String in"=w404) -> ("String out"=w401:string)  [unwired: 6 in, 1 out]
              n118 = call "setKey.vi"("LegendProperties"=w384, "Set?"=w383, "String in"=w401) -> ("String out"=w400:string)  [unwired: 7 in, 1 out]
              n119 = call "AxisControl.vi"("String in"=w400, "AxisBounds"=w381, "ticsAndGrids"=w386, "Axis"=w390, "ShowNumbers?"=w398, "ShowLabel?"=w397, "Axis Label"=w391, "DataSpan"=w380) -> ("String out"=w393:string)  [unwired: 6 in, 1 out]
              n120 = call "AxisControl.vi"("String in"=w393, "AxisBounds"=w382, "ticsAndGrids"=w387, "Axis"=w389, "ShowNumbers?"=w396, "ShowLabel?"=w395, "Axis Label"=w388, "DataSpan"=w379) -> ("String out"=w399:string)  [unwired: 6 in, 1 out]
              n121 = Concatenate Strings(w399, w405) -> (w406:string)
            }
          }
        }
        n122 = Concatenate Strings(w318, w319, "\nunset multiplot\n") -> (w324:string)
      }
      frame "Write gnuplot file" {
        w414 = FALSE  # append to file? (new file:F)
        w415 = FALSE  # advisory dialog? (display:T)
        n123 = Strip Path(path=w411) -> (stripped path=w408:path)  [unwired: 1 out]
        n124 = Build Path(base path=w408, name or relative path="gnuplot_script.txt") -> (appended path=w416:path)
        n125 = call "Write_Characters_To_File.vi"("file path (dialog if empty)"=w416, "advisory dialog? (display:T)"=w415, "character string"=w407, "append to file? (new file:F)"=w414) -> ()  [unwired: 1 in, 4 out]
      }
      frame "Execute shell script" {
        n126 = call "Run_Gnuplot_Script.vi"("logfileName"=w418, "workingDirectory"=w419) -> ()
      }
      frame "Has pdf been generated?" {
        n127 = Select(t="Open Standard output file" ("f"), s="OpenLogfile?", f="End") -> (s? t:f=w425:string)
        n128 = Select(t="Show Re-Run Gnuplot?", s="Show Script Editor?", f=w425) -> (s? t:f=w429:string)
      }
      frame "Show Re-Run Gnuplot?" {
        n129 = Strip Path(path=w438) -> (stripped path=w437:path)  [unwired: 1 out]
        n130 = call "Re_run_Gnuplot.vi"("Plot folder (dialog if empty)"=w437) -> ()  [unwired: 4 out]
      }
      frame "Open Standard output file" {
        n131 = Strip Path(path=w448) -> (stripped path=w445:path)  [unwired: 1 out]
        n132 = Format Into String(format string="open \"%s\"", w446) -> (resulting string=w444:string)  [unwired: 2 in, 1 out]
        n133 = call <vilib>:"System Exec.vi"("working directory"=w445, "command line"=w444) -> ()  [unwired: 4 in, 6 out]
      }
      frame "End" {
      }
    }
    "gnuplotScript" <- w17
  }
  "AuditTrail" <- w4
  "Saved Automatically?" <- FALSE
